vi "试剂余量后台任务.vi"   [LabVIEW 2016, in "斯坦道氨氮.lvlib"]
uses:
  <vilib>/ptbypt/NI_PtbyPt.lvlib
types:
  T1 = cluster{"V1":sgl, "V2":sgl, "V3":sgl, "V4":sgl, "V5":sgl, "V6":sgl, "V7":sgl, "V8":sgl, "V9":sgl, "V10":sgl, "V11":sgl, "V12":sgl, "V9-1":sgl, "V9-2":sgl}
  T2 = cluster{"时间标识":timestamp, "设备":string, "日志信息":string, "备注":string}
  T3 = cluster{"系统时间":timestamp, "工作状态":u16, "测量模式":enum16{"待机", "连续模式", "周期模式", "定点模式", "受控模式", "手动模式"}, "告警代码":u16, "故障代码":u16, "日志代码":u16, "软件版本":u16, "F0":sgl, "F1":sgl, "F2":sgl, "F3":sgl, "T":sgl, "H":sgl, "id":u16, "flowid":u16, "量程":u16, "总磷控温温度1":sgl, "营养盐控温温度2":sgl, "ADC":sgl}
  T4 = cluster{"V1":bool, "V2":bool, "V3":bool, "V4":bool, "V5":bool, "V6":bool, "V7":bool, "V8":bool, "V9":bool, "V10":bool, "V11":bool, "V12":bool, "V9-1":bool, "V9-2":bool}
  T5 = cluster{"参数":string, "报警内容":string, "报警分析":string}
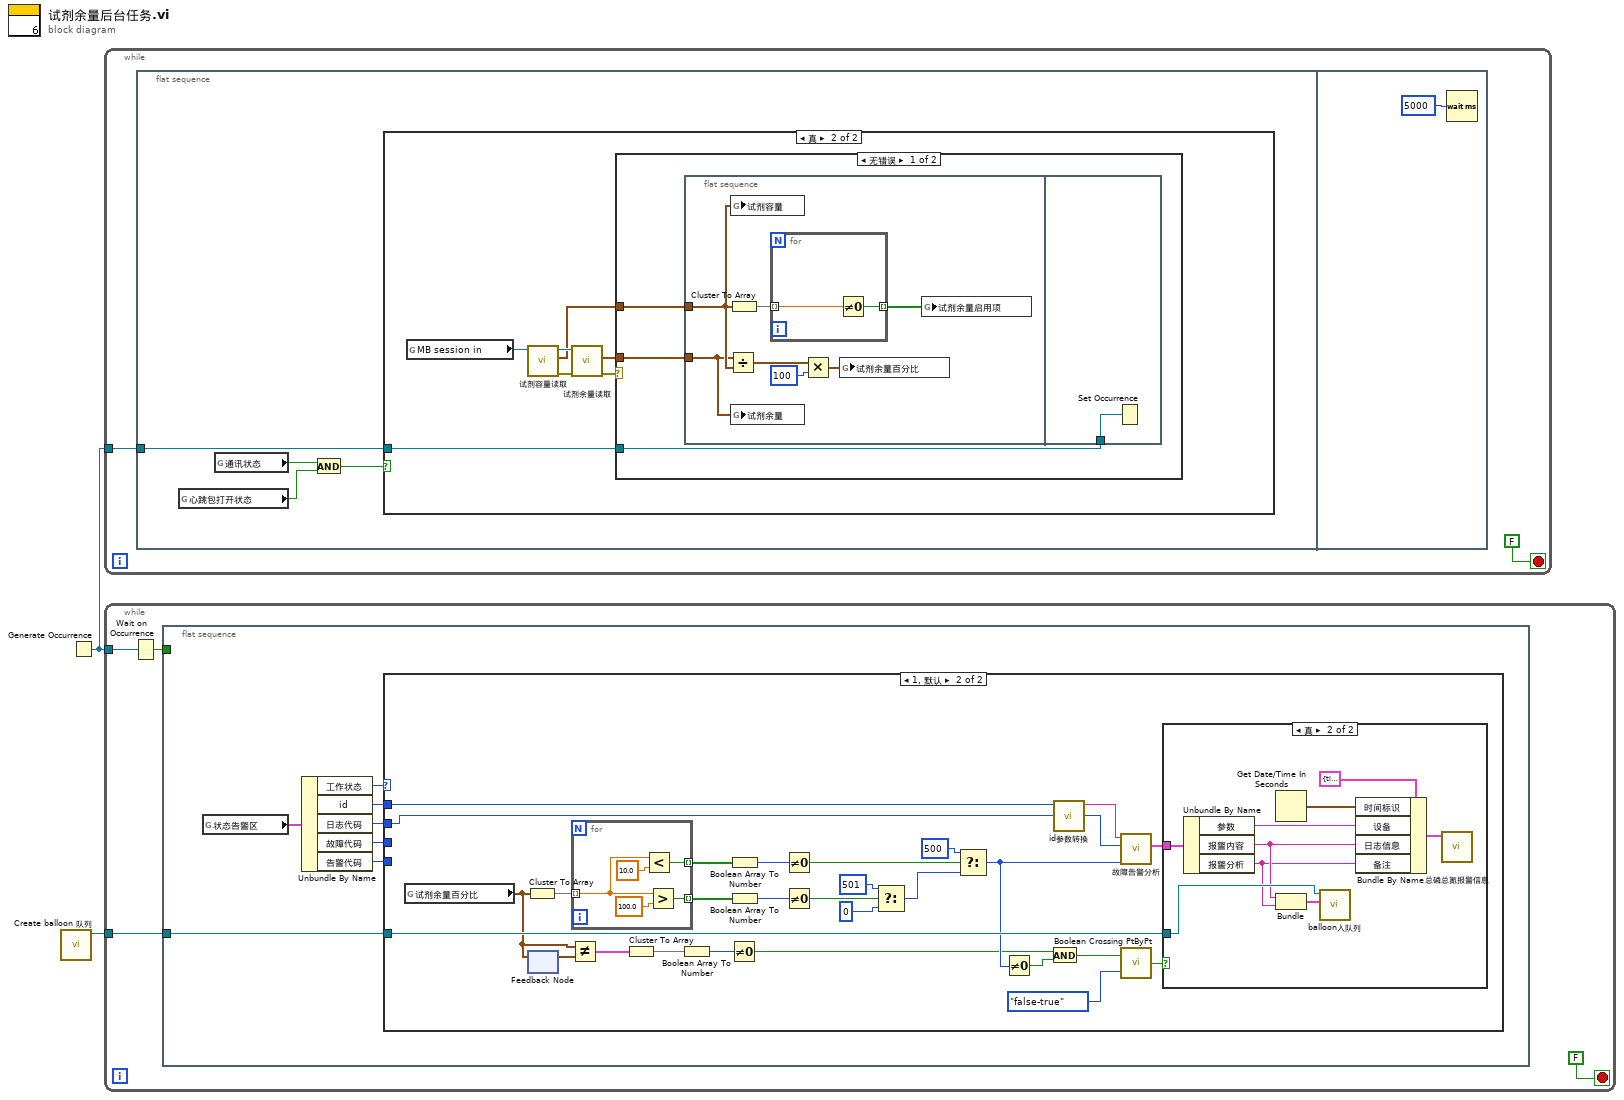
[diagram p0: block diagram]
diagram:
  n1 = call "Create balloon 队列.vi"() -> ("队列输出"=w2:refnum<queue>)  [unwired: 11 in]
  n2 = Generate Occurrence() -> (w1:refnum<k4>)
  n3 = while {
    tunnel: w1 -> [w3]
    stop <- FALSE stop-if-true
    n4 = flat-sequence {
      tunnel: w3 -> [w8]
      frame #0 {
        n5 = global read "VAR总磷总氮全局变量.vi" "心跳包打开状态"() -> (w7:bool)
        n6 = global read "VAR总磷总氮全局变量.vi" "通讯状态"() -> (w5:bool)
        n7 = And(x=w5, y=w7) -> (x .and. y?=w6:bool)
        n8 = case shown="真" w6 {
          tunnel: w8 -> [_ w9]
          frame False {
          }
          frame True {
            n9 = global read "VAR总磷总氮全局变量.vi" "MB session in"() -> (w13:refnum<class "MB_Master.lvclass">)
            n10 = call "试剂容量读取.vi"("MB session in"=w13) -> ("error out"=w15:errorcluster, "试剂容量"=w12:T1, "MB session out"=w14:refnum<class "MB_Master.lvclass">)  [unwired: 8 in]
            n11 = call "试剂余量读取.vi"("Error in"=w15, "MB session in"=w14) -> ("error out"=w10:errorcluster, "试剂余量"=w11:T1)  [unwired: 7 in, 1 out]
            n12 = case shown="无错误" w10 {
              tunnel: w12 -> [w18 _]
              tunnel: w11 -> [w17 _]
              tunnel: w9 -> [w16 _]
              frame No Error {
                n13 = flat-sequence {
                  tunnel: w18 -> [w23]
                  tunnel: w17 -> [w22]
                  tunnel: w16 -> [w28]
                  frame #0 {
                    n14 = Divide(x=w22, y=w23) -> (x/y=w25:T1)
                    n15 = Cluster To Array(cluster=w23) -> (array=w20:sgl[])
                    n16 = global write "VAR总磷总氮全局变量.vi" "试剂容量"(w23) -> ()
                    n17 = global write "VAR总磷总氮全局变量.vi" "试剂余量"(w22) -> ()
                    n18 = for {
                      tunnel: w20 -> [w27] mode=indexing
                      tunnel: [w26] -> w19 mode=indexing
                      n19 = Not Equal To 0?(x=w27) -> (x != 0?=w26:bool)
                    }
                    n20 = Multiply(x=w25, y=100) -> (x*y=w21:T1)
                    n21 = global write "VAR总磷总氮全局变量.vi" "试剂余量百分比"(w21) -> ()
                    n22 = global write "VAR总磷总氮全局变量.vi" "试剂余量启用项"(w19) -> ()
                  }
                  frame #1 {
                    n23 = Set Occurrence(w28) -> ()
                  }
                }
              }
              frame Error {
              }
            }
          }
        }
      }
      frame #1 {
        n24 = Wait (ms)(milliseconds to wait=u32 5000 ("等待时间（毫秒）")) -> ()  [unwired: 1 out]
      }
    }
  }
  n25 = while {
    tunnel: w2 -> [w32]
    tunnel: w1 -> [w31]
    stop <- FALSE stop-if-true
    n26 = Wait on Occurrence(2:w31) -> (0:w30:bool)  [unwired: 2 in]
    n27 = flat-sequence {
      tunnel: w32 -> [w38]
      tunnel: w30 -> [_]
      frame #0 {
        n28 = global read "VAR总磷总氮全局变量.vi" "状态告警区"() -> (w34:T3)
        n29 = Unbundle By Name(w34) -> ("工作状态"=w35:u16, "id"=w40:u16, "日志代码"=w39:u16, "故障代码"=w37:u16, "告警代码"=w36:u16)
        n30 = case shown="1, 默认" w35 {
          tunnel: w40 -> [_ w67]
          tunnel: w39 -> [_ w66]
          tunnel: w38 -> [_ w63]
          tunnel: w37 -> [_ _]
          tunnel: w36 -> [_ _]
          frame 0 {
          }
          frame 1, Default {
            n31 = global read "VAR总磷总氮全局变量.vi" "试剂余量百分比"() -> (w48:T1)
            n32 = Cluster To Array(cluster=w48) -> (array=w58:sgl[])
            n33 = feedback-in #1(w48) -> ()
            n34 = feedback #1() -> (w49:T1)  [unwired: 1 in]
            n35 = Not Equal?(x=w48, y=w49) -> (x != y?=w47:T4)
            n36 = for {
              tunnel: w58 -> [w70] mode=indexing
              tunnel: [w71] -> w60 mode=indexing
              tunnel: [w68] -> w59 mode=indexing
              n37 = Less?(x=w70, y=sgl 10.0) -> (x < y?=w71:bool)
              n38 = Greater?(x=w70, y=sgl 100.0) -> (0:w68:bool)
            }
            n39 = Cluster To Array(cluster=w47) -> (array=w46:bool[])
            n40 = Boolean Array To Number(Boolean array=w46) -> (number=w45:u32)
            n41 = Not Equal To 0?(x=w45) -> (x != 0?=w43:bool)
            n42 = Boolean Array To Number(Boolean array=w60) -> (number=w62:u32)
            n43 = Boolean Array To Number(Boolean array=w59) -> (number=w61:u32)
            n44 = Not Equal To 0?(x=w62) -> (x != 0?=w57:bool)
            n45 = Not Equal To 0?(x=w61) -> (x != 0?=w55:bool)
            n46 = Select(t=501, s=w55, f=0) -> (s? t:f=w52:i32)
            n47 = Select(t=500, s=w57, f=w52) -> (s? t:f=w51:i32)
            n48 = Not Equal To 0?(x=w51) -> (x != 0?=w50:bool)
            n49 = And(x=w43, y=w50) -> (x .and. y?=w44:bool)
            n50 = call "id参数转换.vi"("id"=w67) -> ("table输出"=w64:string)  [unwired: 9 in, 1 out]
            n51 = call "故障告警分析.vi"("告警代码"=w51, "运行步序"=w66, "参数"=w64) -> ("报警内容"=w65:T5)  [unwired: 7 in, 1 out]
            n52 = call <vilib>:"Boolean Crossing PtByPt.vi"("direction"=enum16{"either", "false-true", "true-false"}."false-true", "input"=w44) -> ("crossing"=w42:bool)  [unwired: 1 in]
            n53 = case shown="真" w42 {
              tunnel: w65 -> [_ w81]
              tunnel: w63 -> [_ w80]
              frame False {
              }
              frame True {
                n54 = Unbundle By Name(w81) -> ("参数"=w76:string, "报警内容"=w75:string, "报警分析"=w74:string)
                n55 = Get Date/Time In Seconds() -> (seconds since 1Jan1904=w79:timestamp)
                n56 = Bundle("报警内容"=w75, "报警分析"=w74) -> (w73:cluster{"报警内容":string, "报警分析":string})  [unwired: 1 in]
                n57 = call "balloon入队列.vi"("报警内容"=w73, "队列"=w80) -> ()  [unwired: 9 in, 1 out]
                n58 = Bundle By Name(cluster=T2 {"时间标识"=timestamp(0 s since 1904-01-01), "设备"="", "日志信息"="", "备注"=""} ("data in"), "时间标识"=w79, "设备"=w76, "日志信息"=w75, "备注"=w74) -> (w78:T2)
                n59 = call "总磷总氮报警信息.vi"("data in"=w78) -> ()  [unwired: 10 in, 1 out]
              }
            }
          }
        }
      }
    }
  }
